vi "Take_C1_C2_Then_C1+C2_Shell.vi"(3 "Mode":T5, 5 "Traverse line In":T2 {"Row Duration (mins)" format="%#.1f"; "Row No" min=0; "Trace Gas Concentration (%)" min=0.0 format="%#.2f"; "Emission Rate (l/min)" format="%#.2f"; "Tunnel Speed" format="%#.2f"; "Start X" format="%#.2f"; "Start Y" format="%#.2f"; "Start Z" format="%#.2f"; "End X" format="%#.2f"; "End Y" format="%#.2f"; "End Z" format="%#.2f"; "Averaging time (min)" min=0.0 format="%#.1f"}) -> (0 "Error Message":string, 1 "Status":T1, 2 "Traverse line Out":T2 {"Row Duration (mins)" format="%#.1f"; "Row No" min=0; "Trace Gas Concentration (%)" min=0.0 format="%#.2f"; "Emission Rate (l/min)" format="%#.2f"; "Tunnel Speed" format="%#.2f"; "Start X" format="%#.2f"; "Start Y" format="%#.2f"; "Start Z" format="%#.2f"; "End X" format="%#.2f"; "End Y" format="%#.2f"; "End Z" format="%#.2f"; "Averaging time (min)" min=0.0 format="%#.1f"})   [LabVIEW 2010]
uses:
  Gen Trav/Traverse_cluster.ctl
  Gen Trav/Spacing.ctl
  Controls/Multi_run_mode.ctl
  Controls/User_Specific_mode.ctl
  Gen Trav/Multi_Run_Status.ctl
  Controls/Save_Data.ctl
  Controls/Setup.ctl
  Plug in sub vis/Extra_info.vi
  Globals/Meas_global.vi
panel:
  out "Current Case":string
  out "Ch Values":string[](array[string])
  out "Ch Names":string[](array[string])
  # "X           Y            Z"
  # "Start"
  # "End"
  # "X           Y            Z"
  # "Start"
  # "End"
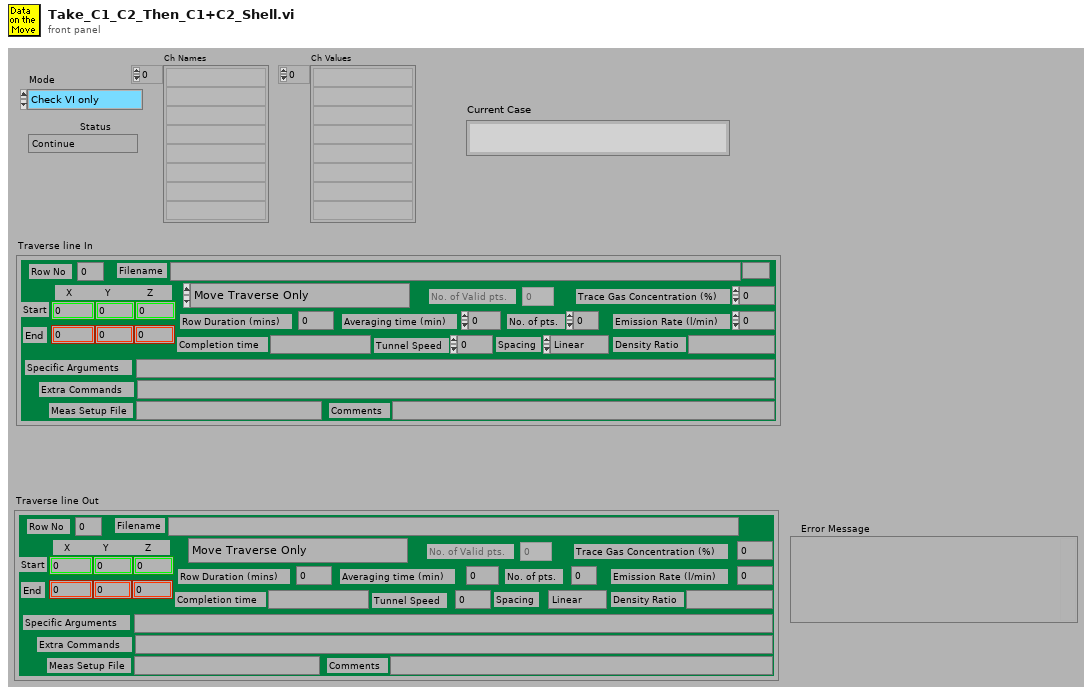
[diagram p1: front panel]
types:
  T1 = typedef "Multi_Run_Status.ctl" = enum16{"Continue", "Jump to Next Point", "Jump to Next Row", "Jump To Fall Back", "Terminate Run"}
  T2 = typedef "Traverse_cluster.ctl" = cluster{"Start X":dbl, "Start Y":dbl, "Start Z":dbl, "End X":dbl, "End Y":dbl, "End Z":dbl, "No. of pts.":i32, "Spacing":T3, "Filename":path, "Tunnel Speed":dbl, "Averaging time (min)":dbl, "Extra Commands":string, "Specific Arguments":string, "Emission Rate (l/min)":dbl, "Trace Gas Concentration (%)":dbl, "Density Ratio":string, "Comments":string, "Row No":i32, "Row Type Selector":T4, "Completion time":string, "Row Duration (mins)":dbl, "No. of Valid pts.":i32, "Meas Setup File":string}
  T3 = typedef "Spacing.ctl" = enum16{"Linear", "Log", "Gauss", "Specified", "N/A"}
  T4 = typedef "Multi_run_mode.ctl" = enum16{"Move Traverse Only", "Set Tunnel Speed Only", "Set Source Only", "Set Measurement Conditions", "Single Measurement", "Vertical Profile", "Lateral Profile", "Longitudinal Profile", "Explore Volume", "Multi-Axis Profile", "Auto Calibrate", "Meas Fast FID Bkgnd", "Check Beam Power", "Scanning Valve Measurement", "Run VI Named:", "Set ADAM Ch", "Wait (minutes)", "Send Message", "Synchronize With:", "Fall Back to this Row", "Turn Off Row Repeating", "Blank Row"}
  T5 = typedef "User_Specific_mode.ctl" = enum16{"Check VI only", "Run VI"}
  T6 = enum16{"Source 1 only", "Source 2 only", "Both Sources"}
  T7 = typedef "Save_Data.ctl" = enum16{"Save No Data", "Save Data"}
  T8 = typedef "Setup.ctl" = enum16{"Run Program", "Show Setup", "Save Current Setup", "Setup Front Panel"}
  T9 = typedef "Status_Cluster.ctl" = cluster{"Status":T1, "Error Type":string, "Error Description":string}
  T10 = typedef "Velocity_cluster.ctl" = cluster{"Name":string, "U":dbl, "u^2":dbl, "u^3/(u^2)^(1.5)":dbl, "u^4/(u^2)^2 -3":dbl, "% u'/U":dbl, "Mean % Err":dbl, "u^4":dbl}
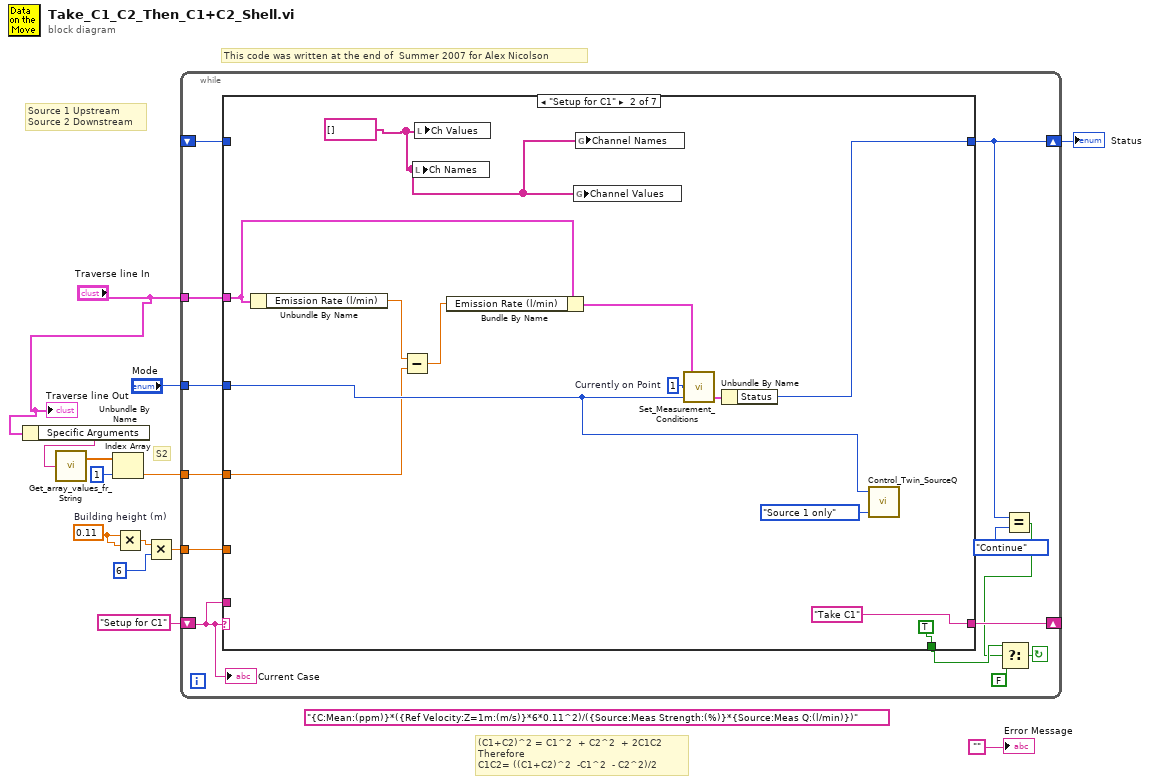
[diagram p0: block diagram]
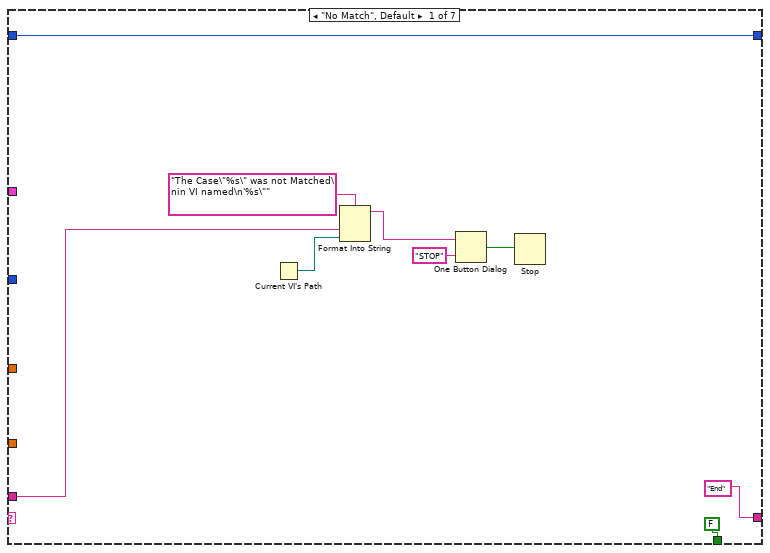
[diagram p2: hidden frame]
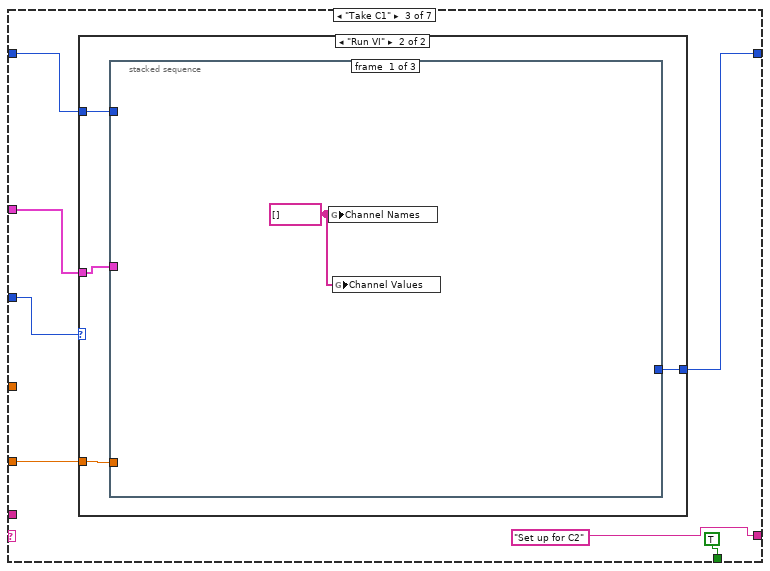
[diagram p3: hidden frame]
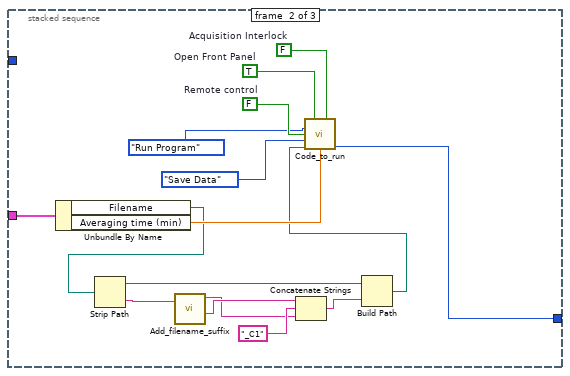
[diagram p5: hidden frame]
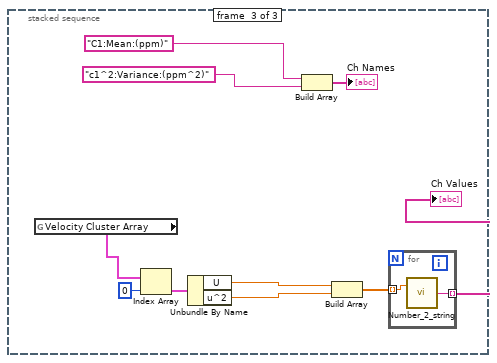
[diagram p6: hidden frame]
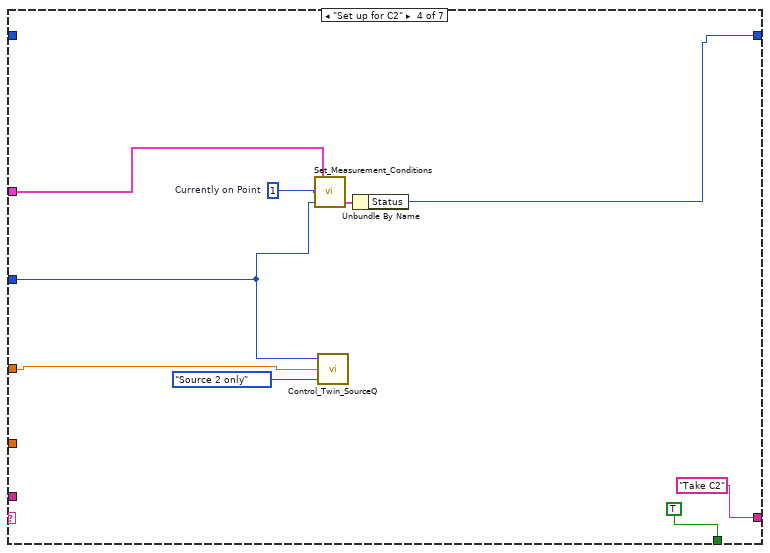
[diagram p7: hidden frame]
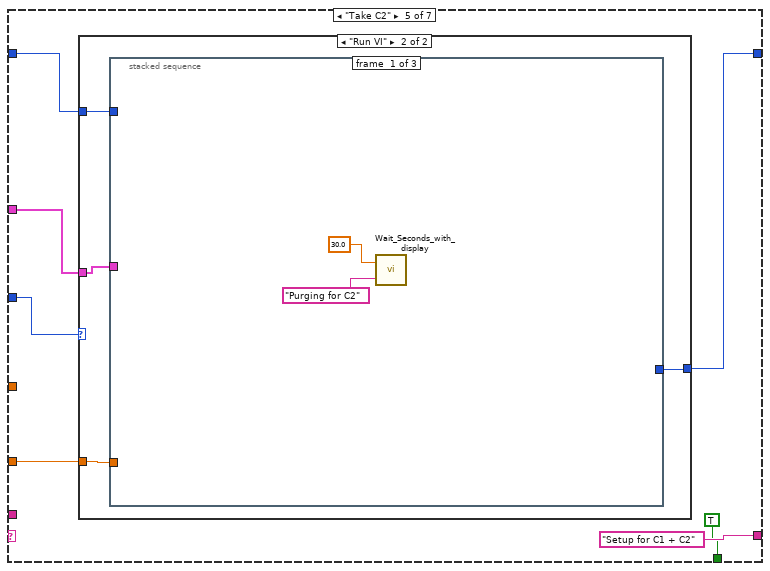
[diagram p8: hidden frame]
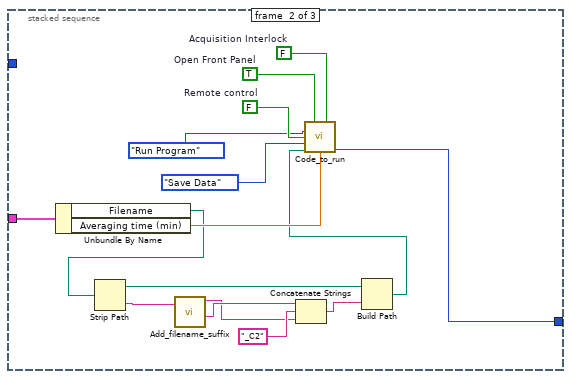
[diagram p10: hidden frame]
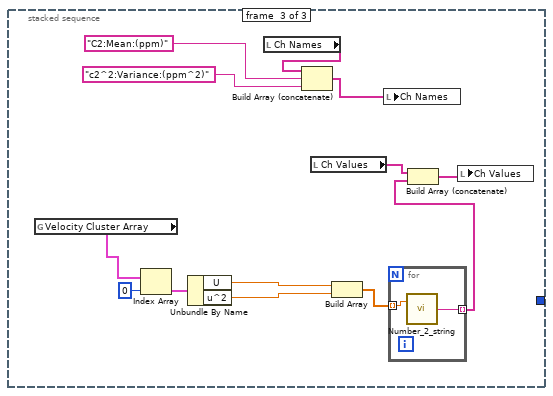
[diagram p11: hidden frame]
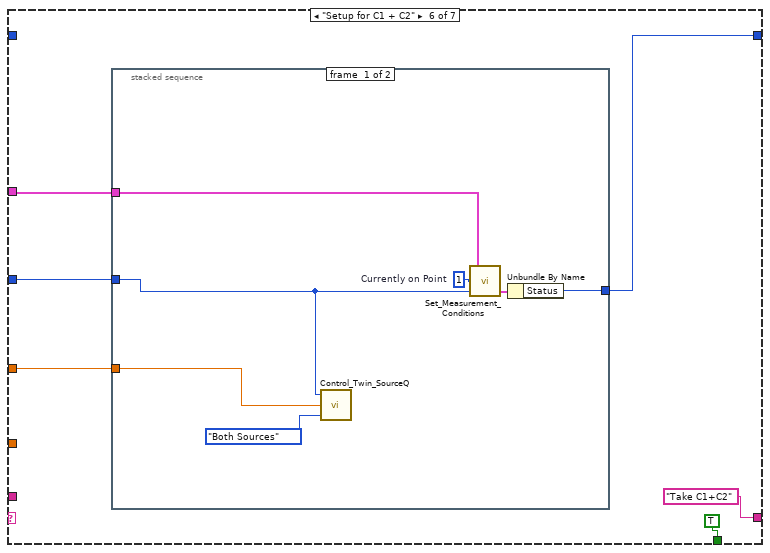
[diagram p12: hidden frame]
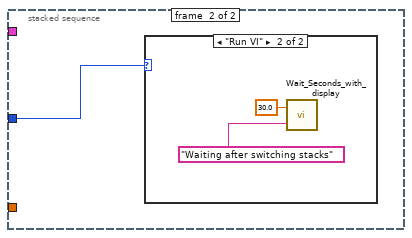
[diagram p13: hidden frame]
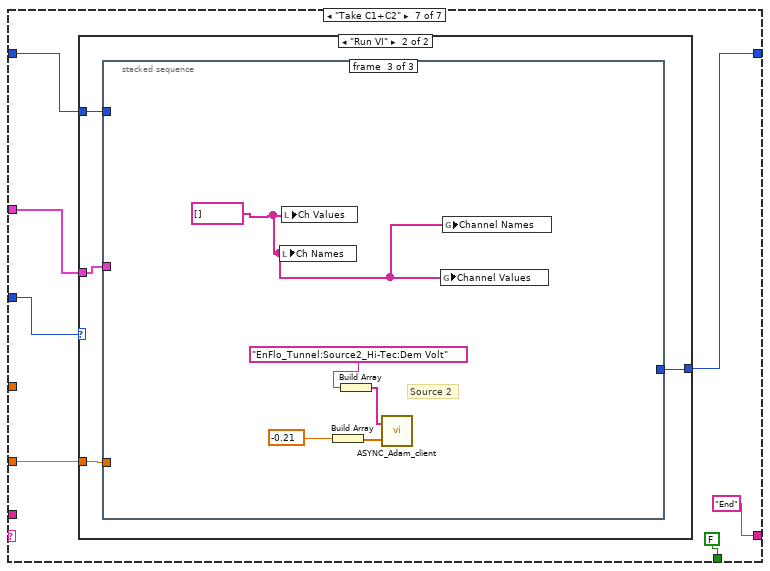
[diagram p15: hidden frame]
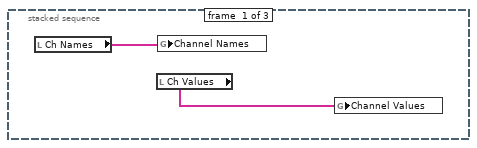
[diagram p17: hidden frame]
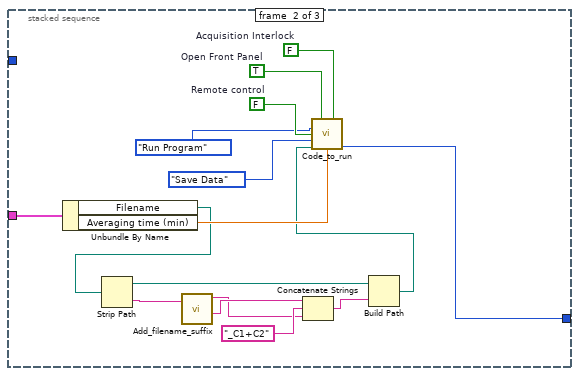
[diagram p18: hidden frame]
diagram:
  w10 = 0.11  # Building height (m)
  (unwired) "{C:Mean:(ppm)}*({Ref Velocity:Z=1m:(m/s)}*6*0.11^2)/({Source:Meas Strength:(%)}*{Source:Meas Q:(l/min)})"
  # "(C1+C2)^2 = C1^2  + C2^2  + 2C1C2\nTherefore\nC1C2= ((C1+C2)^2  -C1^2  - C2^2)/2"
  # "Source 1 Upstream\nSource 2 Downstream"
  # "S2"
  # "This code was written at the end of  Summer 2007 for Alex Nicolson"
  n1 = Unbundle By Name("Traverse line In") -> ("Specific Arguments"=w2:string)
  n2 = call "Get_array_values_fr_String.vi"("String Value"=w2) -> ("Numeric Array"=w4:dbl[])  [unwired: 1 out]
  n3 = Index Array(array=w4, index=1) -> (element=w1:dbl)
  n4 = Multiply(x=w10, y=w10) -> (x*y=w9:dbl)
  n5 = Multiply(x=w9, y=6) -> (x*y=w7:dbl)
  n6 = while {
    shift-left: _ -> [w24]
    shift-right: [w19] -> w11
    tunnel: "Traverse line In" -> [w25]
    tunnel: "Mode" -> [w26]
    shift-left: "Setup for C1" -> [w14]
    shift-right: [w23] -> _
    tunnel: w7 -> [w16]
    tunnel: w1 -> [w15]
    stop <- w17 continue-if-true
    n7 = case shown="\"Setup for C1\"" w14 {
      tunnel: w25 -> [_ w46 w54 w96 w104 w149 w165]
      tunnel: w26 -> [_ w41 w55 w95 w105 w145 w166]
      tunnel: [FALSE ("Update Datum Powers?") TRUE ("Update Datum Powers?") TRUE ("Update Datum Powers?") TRUE ("Update Datum Powers?") TRUE ("Update Datum Powers?") TRUE ("Update Datum Powers?") FALSE ("Update Datum Powers?")] -> w22
      tunnel: ["End" "Take C1" "Set up for C2" "Take C2" "Setup for C1 + C2" "Take C1+C2" "End"] -> w23
      tunnel: w14 -> [w28 _ _ _ _ _ _]
      tunnel: w24 -> [w27 _ w52 _ w102 _ w163]
      tunnel: [w27 w44 w49 w94 w99 w147 w160] -> w19
      tunnel: w16 -> [_ _ w53 _ w103 _ w164]
      tunnel: w15 -> [_ w38 _ w93 _ w144 _]
      frame "No Match", Default {
        n8 = Current VI's Path() -> (path=w31:path)
        n9 = Format Into String(format string="The Case\"%s\" was not Matched\nin VI named\n'%s\"" ("Format String"), w28, w31) -> (resulting string=w34:string)  [unwired: 2 in, 1 out]
        n10 = One Button Dialog(message=w34, button name ("OK")="STOP") -> (true=w32:bool)
        n11 = Stop(stop? (T)=w32) -> ()
      }
      frame "Setup for C1" {
        w40 = string[] [] ("Ch Values")
        w47 = 1  # Currently on Point
        n12 = Unbundle By Name(w46) -> ("Emission Rate (l/min)"=w39:dbl)
        n13 = Subtract(x=w39, y=w38) -> (x-y=w37:dbl)
        n14 = local write "Ch Names"(w40) -> ()
        n15 = local write "Ch Values"(w40) -> ()
        n16 = Bundle By Name(cluster=w46, "Emission Rate (l/min)"=w37) -> (w45:T2)
        n17 = global write "Extra_info.vi" "Channel Values"(w40) -> ()
        n18 = global write "Extra_info.vi" "Channel Names"(w40) -> ()
        n19 = call "Set_Measurement_Conditions.vi"("Simulate/Run"=w41, "Currently on Point"=w47, "Traverse line"=w45) -> ("Status Cluster"=w48:T9)  [unwired: 2 out]
        n20 = Unbundle By Name(w48) -> ("Status"=w44:T1)
        n21 = call "Control_Twin_SourceQ.vi"("Control"=T6."Source 1 only", "Mode"=w41) -> ()  [unwired: 1 in]
      }
      frame "Take C1" {
        n22 = case shown="\"Run VI\"" w55 {
          tunnel: [w56 w60] -> w49
          tunnel: w54 -> [_ w59]
          tunnel: w53 -> [_ w58]
          tunnel: w52 -> [w56 w57]
          frame "Check VI only" {
          }
          frame "Run VI" {
            n23 = stacked-sequence {
              tunnel: [_ w77 _] -> w60
              tunnel: w59 -> [_ w76 _]
              tunnel: w58 -> [_ _ _]
              tunnel: w57 -> [_ _ _]
              frame #0 {
                w61 = string[] [] ("Channel Names")
                n24 = global write "Extra_info.vi" "Channel Names"(w61) -> ()
                n25 = global write "Extra_info.vi" "Channel Values"(w61) -> ()
              }
              frame #1 {
                w72 = FALSE  # Acquisition Interlock
                w73 = TRUE  # Open Front Panel
                w75 = FALSE  # Remote control
                n26 = Unbundle By Name(w76) -> ("Filename"=w63:path, "Averaging time (min)"=w74:dbl)
                n27 = Strip Path(path=w63) -> (stripped path=w64:path, name=w69:string)
                n28 = call "Add_filename_suffix.vi"("Filename"=w69) -> ("Original Suffix"=w66:string, "Base name"=w68:string)  [unwired: 1 in, 2 out]
                n29 = Concatenate Strings(w68, "_C1" ("string"), w66) -> (w65:string)
                n30 = Build Path(base path=w64, name or relative path=w65) -> (appended path=w62:path)
                n31 = call "Code_to_run.vi"("Open Front Panel"=w73, "Acquisition Interlock"=w72, "setup"=Setup."Run Program", "Remote control"=w75, "File"=Save_Data."Save Data", "Results Filename"=w62, "Averaging time (min)"=w74) -> ("Status"=w77:T1)  [unwired: 4 in, 4 out]
              }
              frame #2 {
                n32 = global read "Meas_global.vi" "Velocity Cluster Array"() -> (w87:T10[])
                n33 = Index Array(array=w87, index=0) -> (element=w85:T10)
                n34 = Unbundle By Name(w85) -> ("U"=w81:dbl, "u^2"=w80:dbl)
                n35 = Build Array("C1:Mean:(ppm)", "c1^2:Variance:(ppm^2)") -> (→"Ch Names":string[])
                n36 = Build Array(w81, w80) -> (w79:dbl[])
                n37 = for {
                  tunnel: w79 -> [w89] mode=indexing
                  tunnel: [w88] -> w78 mode=indexing
                  n38 = call "Number_2_string.vi"("number"=w89) -> ("String"=w88:string)  [unwired: 1 in]
                }
                "Ch Values" <- w78
              }
            }
          }
        }
      }
      frame "Set up for C2" {
        w90 = 1  # Currently on Point
        n39 = call "Set_Measurement_Conditions.vi"("Simulate/Run"=w95, "Currently on Point"=w90, "Traverse line"=w96) -> ("Status Cluster"=w91:T9)  [unwired: 2 out]
        n40 = call "Control_Twin_SourceQ.vi"("Control"=T6."Source 2 only" ("Mode"), "Source2 Flowrate l/min"=w93, "Mode"=w95) -> ()
        n41 = Unbundle By Name(w91) -> ("Status"=w94:T1)
      }
      frame "Take C2" {
        n42 = case shown="\"Run VI\"" w105 {
          tunnel: [w106 w110] -> w99
          tunnel: w104 -> [_ w109]
          tunnel: w103 -> [_ w108]
          tunnel: w102 -> [w106 w107]
          frame "Check VI only" {
          }
          frame "Run VI" {
            n43 = stacked-sequence {
              tunnel: [_ w128 _] -> w110
              tunnel: w109 -> [_ w127 _]
              tunnel: w108 -> [_ _ _]
              tunnel: w107 -> [_ _ _]
              frame #0 {
                n44 = call "Wait_Seconds_with_display.vi"("Message"="Purging for C2", "Seconds to wait"=30.0) -> ()  [unwired: 2 out]
              }
              frame #1 {
                w123 = FALSE  # Acquisition Interlock
                w124 = TRUE  # Open Front Panel
                w126 = FALSE  # Remote control
                n45 = Unbundle By Name(w127) -> ("Filename"=w114:path, "Averaging time (min)"=w125:dbl)
                n46 = Strip Path(path=w114) -> (stripped path=w115:path, name=w120:string)
                n47 = call "Add_filename_suffix.vi"("Filename"=w120) -> ("Original Suffix"=w117:string, "Base name"=w119:string)  [unwired: 1 in, 2 out]
                n48 = Concatenate Strings(w119, "_C2" ("string"), w117) -> (w116:string)
                n49 = Build Path(base path=w115, name or relative path=w116) -> (appended path=w113:path)
                n50 = call "Code_to_run.vi"("Open Front Panel"=w124, "Acquisition Interlock"=w123, "setup"=Setup."Run Program", "Remote control"=w126, "File"=Save_Data."Save Data", "Results Filename"=w113, "Averaging time (min)"=w125) -> ("Status"=w128:T1)  [unwired: 4 in, 4 out]
              }
              frame #2 {
                n51 = global read "Meas_global.vi" "Velocity Cluster Array"() -> (w141:T10[])
                n52 = Index Array(array=w141, index=0) -> (element=w139:T10)
                n53 = Unbundle By Name(w139) -> ("U"=w136:dbl, "u^2"=w135:dbl)
                n54 = local read "Ch Names"() -> (w133:string[])
                n55 = Build Array (concatenate)(w133, "C2:Mean:(ppm)", "c2^2:Variance:(ppm^2)") -> (w132:string[])
                n56 = local read "Ch Values"() -> (w131:string[])
                n57 = Build Array(w136, w135) -> (w134:dbl[])
                n58 = local write "Ch Names"(w132) -> ()
                n59 = for {
                  tunnel: w134 -> [w143] mode=indexing
                  tunnel: [w142] -> w130 mode=indexing
                  n60 = call "Number_2_string.vi"("number"=w143) -> ("String"=w142:string)  [unwired: 1 in]
                }
                n61 = Build Array (concatenate)(w131, w130) -> (w129:string[])
                n62 = local write "Ch Values"(w129) -> ()
              }
            }
          }
        }
      }
      frame "Setup for C1 + C2" {
        n63 = stacked-sequence {
          tunnel: w149 -> [w153 _]
          tunnel: [w152 _] -> w147
          tunnel: w145 -> [w151 w157]
          tunnel: w144 -> [w150 _]
          frame #0 {
            w155 = 1  # Currently on Point
            n64 = call "Control_Twin_SourceQ.vi"("Control"=T6."Both Sources" ("Mode"), "Source2 Flowrate l/min"=w150, "Mode"=w151) -> ()
            n65 = call "Set_Measurement_Conditions.vi"("Simulate/Run"=w151, "Currently on Point"=w155, "Traverse line"=w153) -> ("Status Cluster"=w156:T9)  [unwired: 2 out]
            n66 = Unbundle By Name(w156) -> ("Status"=w152:T1)
          }
          frame #1 {
            n67 = case shown="\"Run VI\"" w157 {
              frame "Check VI only" {
              }
              frame "Run VI" {
                n68 = call "Wait_Seconds_with_display.vi"("Message"="Waiting after switching stacks", "Seconds to wait"=30.0) -> ()  [unwired: 2 out]
              }
            }
          }
        }
      }
      frame "Take C1+C2" {
        n69 = case shown="\"Run VI\"" w166 {
          tunnel: [w167 w171] -> w160
          tunnel: w165 -> [_ w170]
          tunnel: w164 -> [_ w169]
          tunnel: w163 -> [w167 w168]
          frame "Check VI only" {
          }
          frame "Run VI" {
            n70 = stacked-sequence {
              tunnel: [_ w189 _] -> w171
              tunnel: w170 -> [_ w188 _]
              tunnel: w169 -> [_ _ _]
              tunnel: w168 -> [_ _ _]
              frame #0 {
                n71 = local read "Ch Names"() -> (w173:string[])
                n72 = local read "Ch Values"() -> (w172:string[])
                n73 = global write "Extra_info.vi" "Channel Names"(w173) -> ()
                n74 = global write "Extra_info.vi" "Channel Values"(w172) -> ()
              }
              frame #1 {
                w184 = FALSE  # Acquisition Interlock
                w185 = TRUE  # Open Front Panel
                w187 = FALSE  # Remote control
                n75 = Unbundle By Name(w188) -> ("Filename"=w175:path, "Averaging time (min)"=w186:dbl)
                n76 = Strip Path(path=w175) -> (stripped path=w176:path, name=w181:string)
                n77 = call "Add_filename_suffix.vi"("Filename"=w181) -> ("Original Suffix"=w178:string, "Base name"=w180:string)  [unwired: 1 in, 2 out]
                n78 = Concatenate Strings(w180, "_C1+C2" ("string"), w178) -> (w177:string)
                n79 = Build Path(base path=w176, name or relative path=w177) -> (appended path=w174:path)
                n80 = call "Code_to_run.vi"("Open Front Panel"=w185, "Acquisition Interlock"=w184, "setup"=Setup."Run Program", "Remote control"=w187, "File"=Save_Data."Save Data", "Results Filename"=w174, "Averaging time (min)"=w186) -> ("Status"=w189:T1)  [unwired: 4 in, 4 out]
              }
              frame #2 {
                w194 = string[] [] ("Ch Values")
                # "Source 2"
                n81 = local write "Ch Names"(w194) -> ()
                n82 = local write "Ch Values"(w194) -> ()
                n83 = Build Array(-0.21 ("f")) -> (w191:dbl[])
                n84 = Build Array("EnFlo_Tunnel:Source2_Hi-Tec:Dem Volt") -> (w193:string[])
                n85 = call "ASYNC_Adam_client.vi"("Values"=w191, "Channel Names"=w193) -> ()  [unwired: 2 out]
                n86 = global write "Extra_info.vi" "Channel Values"(w194) -> ()
                n87 = global write "Extra_info.vi" "Channel Names"(w194) -> ()
              }
            }
          }
        }
      }
    }
    n88 = Equal?(x=w19, y=Multi_Run_Status."Continue" ("Status")) -> (x = y?=w21:bool)
    n89 = Select(t=w22, s=w21, f=FALSE) -> (s? t:f=w17:bool)
    "Current Case" <- w14
  }
  "Status" <- w11
  "Error Message" <- ""
  "Traverse line Out" <- "Traverse line In"
